vi "TCP-Init.vi"(11 "error in (no error)":errorcluster) -> (15 "error out":errorcluster)   [LabVIEW 2015]
uses:
  <vilib>/Utility/config.llb/Read Key (String).vi
  DAQ Engine VIs/PXI Globals.vi
  <vilib>/Utility/config.llb/NI_LVConfig.lvlib
panel:
  out "Client":string
  out "Server":string
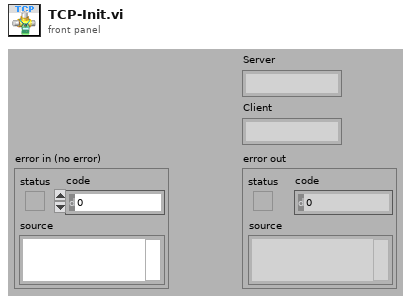
[diagram p1: front panel]
types:
  T1 = typedef "NI_LVConfig.lvlib/Config Data RefNum.ctl" = refnum<k1>
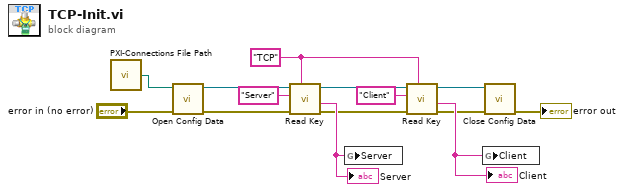
[diagram p0: block diagram]
diagram:
  w7 = "TCP" ("section")
  n1 = call "PXI-Connections File Path.vi"() -> ("Path"=w1:path)  [unwired: 1 in]
  n2 = call <vilib>:"Open Config Data.vi"("error in (no error)"="error in (no error)", "configuration file path"=w1) -> ("error out"=w12:errorcluster, "refnum"=w13:T1)  [unwired: 7 in, 1 out]
  n3 = call-poly <vilib>:"Read Key.vi"("section"=w7, "error in (no error)"=w12, "key"="Server", "refnum"=w13) -> ("error out"=w9:errorcluster, "value"=w10:string, "refnum out"=w8:T1)  [unwired: 4 in, 1 out]
  "Server" <- w10
  n4 = global write "PXI Globals.vi" "Server"(w10) -> ()
  n5 = call-poly <vilib>:"Read Key.vi"("section"=w7, "error in (no error)"=w9, "key"="Client", "refnum"=w8) -> ("error out"=w4:errorcluster, "value"=w5:string, "refnum out"=w3:T1)  [unwired: 4 in, 1 out]
  "Client" <- w5
  n6 = global write "PXI Globals.vi" "Client"(w5) -> ()
  n7 = call <vilib>:"Close Config Data.vi"("error in (no error)"=w4, "refnum"=w3) -> ("error out"=→"error out":errorcluster)  [unwired: 8 in, 1 out]
